vi "Accel_Open.vi"(0 "DIO Module":T3=enum."Digital Module 2", 1 "Range":T1 items=["+/- 2 g"=0, "+/- 4 g"=16, "+/- 8 g"=96], 3 "error in (no error)":errorcluster) -> (7 "I2CDevRef":T2 {"Device Address" format="%.0x"}, 10 "error out":errorcluster)   [LabVIEW 2011]
uses:
  <vilib>/Rock Robotics/SystemInterfaces/Typedef/FPGA_TypedefDigitalModule.ctl
  <vilib>/Rock Robotics/WPI/I2C/WPI_I2CDevRef.ctl
  Accel_Range.ctl
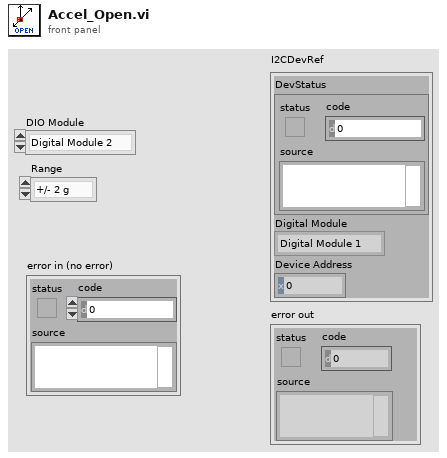
[diagram p1: front panel]
types:
  T1 = typedef "Accel_Range.ctl" = u8
  T2 = typedef "WPI_I2CDevRef.ctl" = cluster{"DevStatus":errorcluster, "Digital Module":T3, "Device Address":u8}
  T3 = typedef "FPGA_TypedefDigitalModule.ctl" = enum16{"Digital Module 1", "Digital Module 2"}
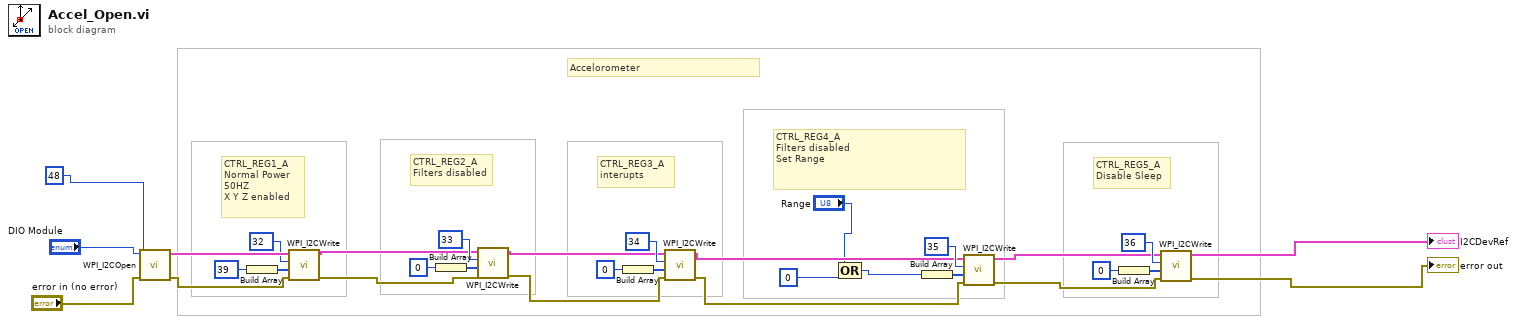
[diagram p0: block diagram]
diagram:
  # "Accelorometer"
  # "CTRL_REG5_A\nDisable Sleep"
  # "CTRL_REG4_A\nFilters disabled\nSet Range"
  # "CTRL_REG3_A\ninterupts"
  # "CTRL_REG2_A\nFilters disabled"
  # "CTRL_REG1_A\nNormal Power \n50HZ\nX Y Z enabled"
  n1 = call <vilib>:"WPI_I2COpen.vi"("error in (no error)"="error in (no error)", "Device Address"=u8 48, "Digital Module (Module 1)"="DIO Module") -> ("error out"=w6:errorcluster, "I2CDevRef"=w31:T2)  [unwired: 7 out]
  n2 = Build Array(u8 39 ("Data To Send")) -> (w28:u8[])
  n3 = call <vilib>:"WPI_I2CWrite.vi"("error in (no error)"=w6, "I2CDataToSend"=w28, "I2CRegister"=u8 32 ("Data To Send"), "I2CDevRef"=w31) -> ("error out"=w5:errorcluster, "I2CDevRef"=w23:T2)  [unwired: 1 in, 5 out]
  n4 = Build Array(u8 0 ("Data To Send")) -> (w24:u8[])
  n5 = call <vilib>:"WPI_I2CWrite.vi"("error in (no error)"=w5, "I2CDataToSend"=w24, "I2CRegister"=u8 33 ("Data To Send"), "I2CDevRef"=w23) -> ("error out"=w4:errorcluster, "I2CDevRef"=w18:T2)  [unwired: 1 in, 5 out]
  n6 = Build Array(u8 0 ("Data To Send")) -> (w20:u8[])
  n7 = call <vilib>:"WPI_I2CWrite.vi"("error in (no error)"=w4, "I2CDataToSend"=w20, "I2CRegister"=u8 34 ("Data To Send"), "I2CDevRef"=w18) -> ("error out"=w3:errorcluster, "I2CDevRef"=w17:T2)  [unwired: 1 in, 5 out]
  n8 = Compound Arithmetic op=OR("Range", u8 0 ("Data To Send")) -> (w10:T1)
  n9 = Build Array(w10) -> (w9:T1[])
  n10 = call <vilib>:"WPI_I2CWrite.vi"("error in (no error)"=w3, "I2CDataToSend"=w9, "I2CRegister"=u8 35 ("Data To Send"), "I2CDevRef"=w17) -> ("error out"=w2:errorcluster, "I2CDevRef"=w13:T2)  [unwired: 1 in, 5 out]
  n11 = Build Array(u8 0 ("Data To Send")) -> (w14:u8[])
  n12 = call <vilib>:"WPI_I2CWrite.vi"("error in (no error)"=w2, "I2CDataToSend"=w14, "I2CRegister"=u8 36 ("Data To Send"), "I2CDevRef"=w13) -> ("error out"=→"error out":errorcluster, "I2CDevRef"=→"I2CDevRef":T2)  [unwired: 1 in, 5 out]
